vi "Shutdown.vi"(8 "error in (no error)":errorcluster, 11 "device data model in":refnum<class "WebSocket Data Model.lvclass">) -> (0 "error out":errorcluster)   [LabVIEW 2021, in "WebSockets.lvlib" / "WebSocket Data Model.lvclass"]
doc: "This VI is responsible for deleting the device data model."
uses:
  WebSocket Data Model.lvclass
  WebSocket Data Model.lvclass/WebSocket Data Model.ctl
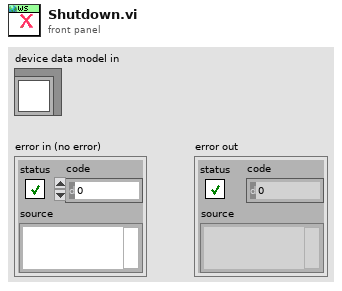
[diagram p1: front panel]
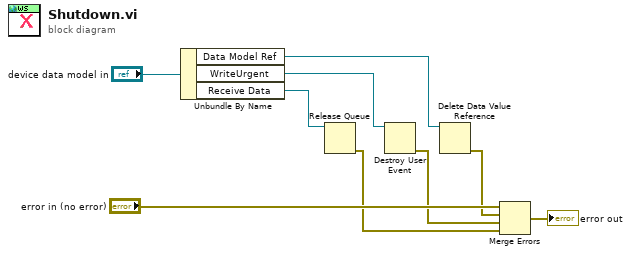
[diagram p0: block diagram]
diagram:
  n1 = Unbundle By Name("device data model in") -> ("Data Model Ref"=w8:refnum<data-value>, "WriteUrgent"=w5:refnum<user-event>, "Receive Data"=w2:refnum<queue>)
  n2 = Release Queue(queue=w2) -> (error out=w1:errorcluster)  [unwired: 2 in, 2 out]
  n3 = Destroy User Event(user event=w5) -> (error out=w3:errorcluster)  [unwired: 1 in]
  n4 = Delete Data Value Reference(data value reference=w8) -> (error out=w4:errorcluster)  [unwired: 1 in, 1 out]
  n5 = Merge Errors("error in (no error)", w4, w3, w1) -> (→"error out":errorcluster)
